vi "test_TranslateLVSymbolicTokenToPath.vi"() -> (3 "Pass?":bool)   [LabVIEW 2019, in "Tests.Utility.lvlib"]
uses:
  Tests.Utility.lvlib
  94cbfa5b-04b5-4af6-9172-05c9669c84fa.vi
  afa44413-be99-4cb9-b869-d5132a8b0d4e.vi
  f25ce0fd-1b01-4f8a-b40c-f219115a22d6.vi
  bda11d55-3d1e-40a5-a186-4b51c9249efc.vi
  3667a24b-cd52-4924-a5e2-285d41a54ba3.vi
  b3525ffb-a664-4abf-9971-66a58ddd2501.vi
  f822f910-59aa-4efb-9f34-1fcce2e2ba81.vi
  59d2ba64-e1ac-41cc-a860-0ca199ca1257.vi
panel:
  out "test results":u32 format="%08b"
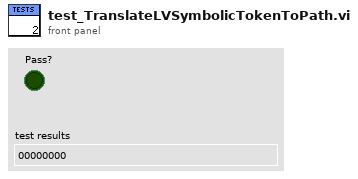
[diagram p1: front panel]
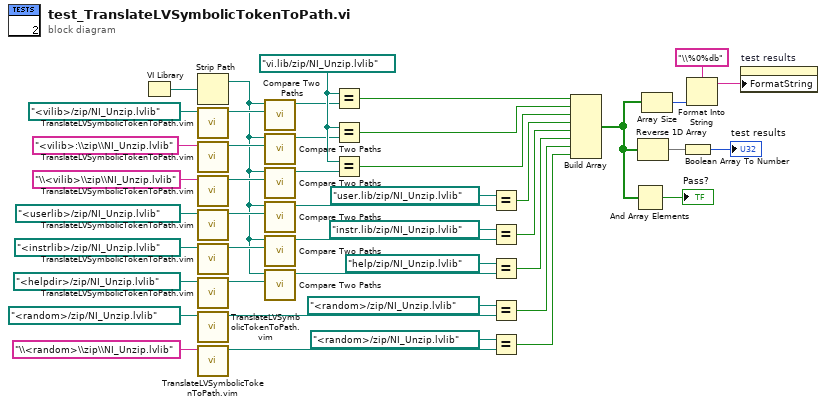
[diagram p0: block diagram]
diagram:
  w35 = path "vi.lib/zip/NI_Unzip.lvlib" ("x")
  n1 = VI Library() -> (path=w28:path)
  n2 = Strip Path(path=w28) -> (stripped path=w21:path)  [unwired: 1 out]
  n3 = call "TranslateLVSymbolicTokenToPath.vim"("Path in"=path "<vilib>/zip/NI_Unzip.lvlib") -> ("Path"=w27:path)  [unwired: 10 in]
  n4 = call "TranslateLVSymbolicTokenToPath.vim"("Path in"="<vilib>:\\zip\\NI_Unzip.lvlib") -> ("Path"=w26:path)  [unwired: 10 in]
  n5 = call "TranslateLVSymbolicTokenToPath.vim"("Path in"="\\<vilib>\\zip\\NI_Unzip.lvlib") -> ("Path"=w25:path)  [unwired: 10 in]
  n6 = call "TranslateLVSymbolicTokenToPath.vim"("Path in"=path "<userlib>/zip/NI_Unzip.lvlib") -> ("Path"=w24:path)  [unwired: 10 in]
  n7 = call "TranslateLVSymbolicTokenToPath.vim"("Path in"=path "<instrlib>/zip/NI_Unzip.lvlib") -> ("Path"=w23:path)  [unwired: 10 in]
  n8 = call "TranslateLVSymbolicTokenToPath.vim"("Path in"=path "<helpdir>/zip/NI_Unzip.lvlib") -> ("Path"=w22:path)  [unwired: 10 in]
  n9 = call "TranslateLVSymbolicTokenToPath.vim"("Path in"=path "<random>/zip/NI_Unzip.lvlib") -> ("Path"=w6:path)  [unwired: 10 in]
  n10 = call "TranslateLVSymbolicTokenToPath.vim"("Path in"="\\<random>\\zip\\NI_Unzip.lvlib") -> ("Path"=w2:path)  [unwired: 10 in]
  n11 = call <vilib>:"Compare Two Paths.vi"("Path 2"=w27, "Path 1"=w21) -> ("Relative Path from 1 to 2"=w20:path)  [unwired: 6 in, 3 out]
  n12 = call <vilib>:"Compare Two Paths.vi"("Path 2"=w26, "Path 1"=w21) -> ("Relative Path from 1 to 2"=w19:path)  [unwired: 6 in, 3 out]
  n13 = call <vilib>:"Compare Two Paths.vi"("Path 2"=w25, "Path 1"=w21) -> ("Relative Path from 1 to 2"=w18:path)  [unwired: 6 in, 3 out]
  n14 = call <vilib>:"Compare Two Paths.vi"("Path 2"=w24, "Path 1"=w21) -> ("Relative Path from 1 to 2"=w17:path)  [unwired: 6 in, 3 out]
  n15 = call <vilib>:"Compare Two Paths.vi"("Path 2"=w23, "Path 1"=w21) -> ("Relative Path from 1 to 2"=w14:path)  [unwired: 6 in, 3 out]
  n16 = call <vilib>:"Compare Two Paths.vi"("Path 2"=w22, "Path 1"=w21) -> ("Relative Path from 1 to 2"=w12:path)  [unwired: 6 in, 3 out]
  n17 = Equal?(x=w35, y=w20) -> (x = y?=w34:bool)
  n18 = Equal?(x=w35, y=w19) -> (x = y?=w33:bool)
  n19 = Equal?(x=w35, y=w18) -> (x = y?=w32:bool)
  n20 = Equal?(x=path "user.lib/zip/NI_Unzip.lvlib", y=w17) -> (x = y?=w11:bool)
  n21 = Equal?(x=path "instr.lib/zip/NI_Unzip.lvlib", y=w14) -> (x = y?=w10:bool)
  n22 = Equal?(x=path "help/zip/NI_Unzip.lvlib", y=w12) -> (x = y?=w9:bool)
  n23 = Equal?(x=path "<random>/zip/NI_Unzip.lvlib", y=w6) -> (x = y?=w5:bool)
  n24 = Equal?(x=path "<random>/zip/NI_Unzip.lvlib", y=w2) -> (x = y?=w1:bool)
  n25 = Build Array(w34, w33, w32, w11, w10, w9, w5, w1) -> (w43:bool[])
  n26 = And Array Elements(Boolean array=w43) -> (logical AND=→"Pass?":bool)
  n27 = Reverse 1D Array(array=w43) -> (reversed array=w39:bool[])
  n28 = Array Size(array=w43) -> (size(s)=w41:i32)
  n29 = Boolean Array To Number(Boolean array=w39) -> (number=→"test results":u32)
  n30 = Format Into String(format string="\\%0%db", w41) -> (resulting string=w40:string)  [unwired: 2 in, 1 out]
  n31 = property on="test results" class="DigNum (strict)"("FormatString"=w40) -> ()  [unwired: 2 in, 2 out]
